vi "Microscope software version global.vi"() -> ()   [LabVIEW 2016]
panel:
  in  "Version String":string="Version 32  (5/18)"
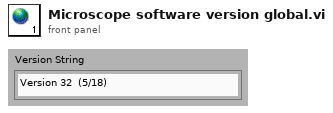
[diagram p1: front panel]
diagram:
